vi "Dialog for DAQmx Configuration.vi"(6 "Variant":variant, 8 "error in":errorcluster, 11 "DAQmx config in":T4={"Run Mode"=0, "Sample Rate (Hz)"=51200.0, "Block Size"=5120, "Channel Table"=[], "Trigger Type"=0, "Trigger Channel"="", "Level"=0.0, "Pretrigger"=20, "Hysteresis"=0.0, "Slope"=enum."Rising"} {"Run Mode" items=["Run Once", "Continuously"]; "Block Size" min=0; "Sample Rate (Hz)" min=0.0; "Trigger Type" items=["None", "Analog Reference"]; "Channel Table"."input terminal configuration" items=["default"=-1, "RSE"=10083, "NRSE"=10078, "Differential"=10106, "Pseudodifferential"=12529]; "Channel Table"."Channel Type" items=["Voltage (V)"=0, "Charge (C)"=9, "-"=99, "SPL (Pa)"=3, "Force (lbf)"=6, "Force (N)"=1, "Acceleration (g) - IEPE"=2, "Acceleration (g) - Charge"=12, "Acceleration (g) - 4 wire DC Voltage"=22, "Velocity (in/s)"=7, "Velocity (mm/s)"=8, "Prox Probe (mil)"=4, "Prox Probe (mm)"=5]}) -> (0 "error out":errorcluster, 1 "Task Verified":T5, 3 "DAQmx config out":T4={"Run Mode"=0, "Sample Rate (Hz)"=51200.0, "Block Size"=5120, "Channel Table"=[], "Trigger Type"=0, "Trigger Channel"="", "Level"=0.0, "Pretrigger"=20, "Hysteresis"=0.0, "Slope"=enum."Rising"} {"Run Mode" items=["Run Once", "Continuously"]; "Block Size" min=0; "Sample Rate (Hz)" min=0.0; "Trigger Type" items=["None", "Analog Reference"]; "Channel Table"."input terminal configuration" items=["default"=-1, "RSE"=10083, "NRSE"=10078, "Differential"=10106, "Pseudodifferential"=12529]; "Channel Table"."Channel Type" items=["Voltage (V)"=0, "Charge (C)"=9, "-"=99, "SPL (Pa)"=3, "Force (lbf)"=6, "Force (N)"=1, "Acceleration (g) - IEPE"=2, "Acceleration (g) - Charge"=12, "Acceleration (g) - 4 wire DC Voltage"=22, "Velocity (in/s)"=7, "Velocity (mm/s)"=8, "Prox Probe (mil)"=4, "Prox Probe (mm)"=5]}, 4 "commit changes":bool)   [LabVIEW 2024, in "Dynamic Signal Acquisition (Interactive) UI.lvlib"]
doc: "Window Appearance = Dialog\n\nThis dialog configuration window reconfigures the DAQmx analog input task."
uses:
  Dynamic Signal Acquisition (Interactive) UI.lvlib
  SFPDAQmx Channel Info.ctl
  SFPDAQ Configuration.ctl
  <vilib>/addons/Sound and Vibration/svt_DAQmx/subVIs/Run Mode.ctl
  <vilib>/addons/Sound and Vibration/svt_DAQmx/subVIs/Verification Status.ctl
  <vilib>/addons/Sound and Vibration/svt_DAQmx/subVIs/Calibration and Reset Status.ctl
  <vilib>/Utility/miscctls.llb/LVPositionTypeDef.ctl
  <vilib>/addons/_NISVFA/_Shared subVIs/Controls/svc_Analog Level Trigger Configuration.ctl
  <vilib>/DAQmx/configure/task.llb/DAQmx Stop Task.vi
  <vilib>/addons/Sound and Vibration/svt_DAQmx/subVIs/Self Calibrate Devices (Dialog).vi
  <vilib>/Utility/cursorutil.llb/Set Busy.vi
  <vilib>/addons/Sound and Vibration/svt_DAQmx/subVIs/Reset Devices.vi
  <vilib>/Utility/cursorutil.llb/Unset Busy.vi
  <vilib>/DAQmx/configure/task.llb/DAQmx Control Task.vi
  <vilib>/addons/_NISVFA/_Shared subVIs/Common/svc_Clear Error Cluster for Specific Code.vi
  <vilib>/addons/Sound and Vibration/svt_DAQmx/subVIs/SV_DAQmx.lvlib
panel:
  in  "Run Mode":T1 items=["Once", "Continuously"]
  in  "Resolution":dbl=10.0 min=0.01 format="%_4g Hz"
  in  "Alias-Free Lines":i32=2000 min=2 max=4000000 step=1 format="%.0f lines"
  in  "Max Frequency":dbl=20000.0 min=0.0 format="%#_g Hz"
  in  "Block Duration":dbl=0.1 min=1e-06 max=100.0 format="%_4g s"
  in  "Block Size":i32=5120 min=2 max=10000000 step=1 format="%.0f samples"
  in  "Sample Rate":dbl=51200.0 min=0.0 format="%#_g Hz"
  in  "Channel Table":T2[](array[typedef]) {"input terminal configuration" items=["default"=-1, "RSE"=10083, "NRSE"=10078, "Differential"=10106, "Pseudodifferential"=12529]; "Channel Type" items=["Voltage (V)"=0, "Charge (C)"=9, "-"=99, "SPL (Pa)"=3, "Force (lbf)"=6, "Force (N)"=1, "Acceleration (g) - IEPE"=2, "Acceleration (g) - Charge"=12, "Acceleration (g) - 4 wire DC Voltage"=22, "Velocity (in/s)"=7, "Velocity (mm/s)"=8, "Prox Probe (mil)"=4, "Prox Probe (mm)"=5]}
  out "status string":string
  out "status":T3
  in  "Reset Devices":bool
  in  "Self Calibrate":bool
  in  "OK":bool
  in  "Error Details":bool
  in  "Cancel":bool
  in  "Slope":enum16{"Falling", "Rising"}(ring)=enum."Rising"
  in  "Hysteresis":dbl format="%#_g EU"
  in  "Pretrigger":i32=20 min=0 step=1 format="%.0f samples"
  in  "Level":dbl format="%#_g EU"
  in  "Channel":string(combo)
  in  "Enable SW Analog Ref Trig":bool
  # "Sampling Info"
  # "Channel Table"
  # "Physical Channel"
  # "Measurement Type"
  # "Range"
  # "mV/EU"
  # "Excitation"
  # "Coupling"
  # "Terminal Configuration"
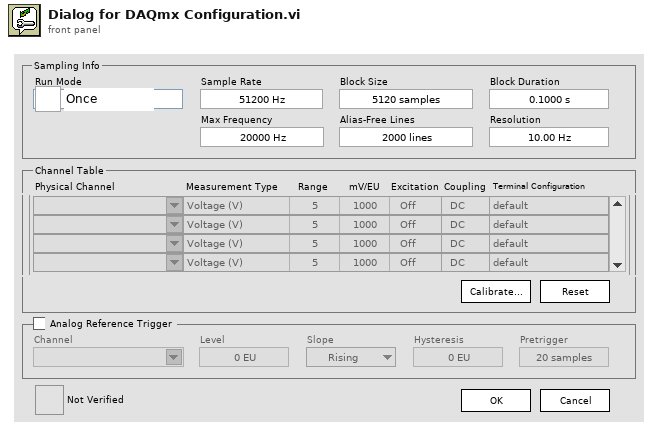
[diagram p1: front panel]
types:
  T1 = typedef "SV_DAQmx.lvlib/Run Mode.ctl" = u16
  T2 = typedef "Dynamic Signal Acquisition (Interactive) UI.lvlib/SFPDAQmx Channel Info.ctl" = cluster{"DAQmx Channel":tag, "Channel Type":u16, "Max":dbl, "Sensitivity":dbl, "Coupling":enum16{"AC", "DC"}, "input terminal configuration":i32, "excitation":enum16{"Off", "Min", "Max"}}
  T3 = typedef "SV_DAQmx.lvlib/Calibration and Reset Status.ctl" = u16
  T4 = typedef "Dynamic Signal Acquisition (Interactive) UI.lvlib/SFPDAQ Configuration.ctl" = cluster{"Run Mode":u16, "Sample Rate (Hz)":dbl, "Block Size":i32, "Channel Table":T2[], "Trigger Type":u16, "Trigger Channel":string, "Level":dbl, "Pretrigger":i32, "Hysteresis":dbl, "Slope":enum16{"Falling", "Rising"}}
  T5 = typedef "SV_DAQmx.lvlib/Verification Status.ctl" = bool
  T6 = enum32{"Invalid", "Standard", "Closed", "Hidden", "Minimized", "Maximized"}
  T7 = typedef "LVPositionTypeDef.ctl" = cluster{"Left":i32, "Top":i32}
  T8 = typedef "LVRectTypeDef.ctl" = cluster{"Left":i16, "Top":i16, "Right":i16, "Bottom":i16}
  T9 = enum8{"Enabled", "Disabled", "Disabled and Grayed Out"}
  T10 = typedef "svc_Analog Level Trigger Configuration.ctl" = cluster{"level":dbl, "slope":u16, "hysteresis":dbl}
  T11 = cluster{"enable":bool, "channel":string, "level trigger configuration":T10, "pretrigger":i32}
  T12 = cluster{"Shift":bool, "Ctrl":bool, "Alt":bool, "Cmd":bool, "Opt":bool}
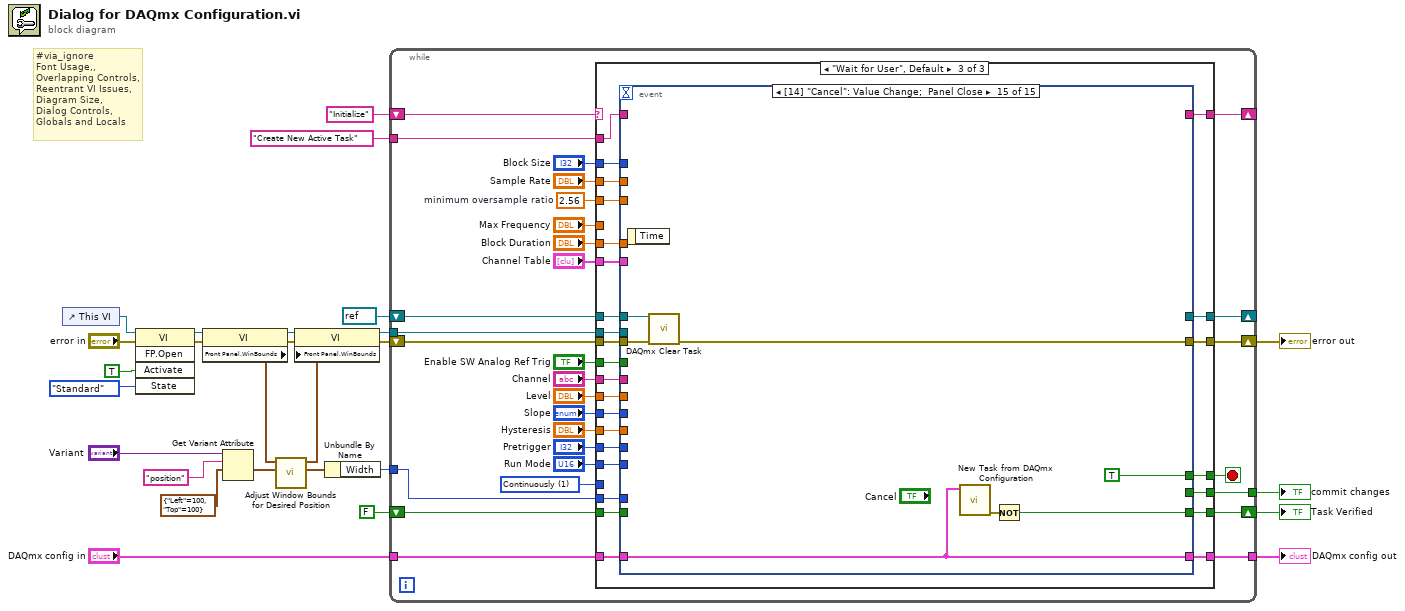
[diagram p0: block diagram]
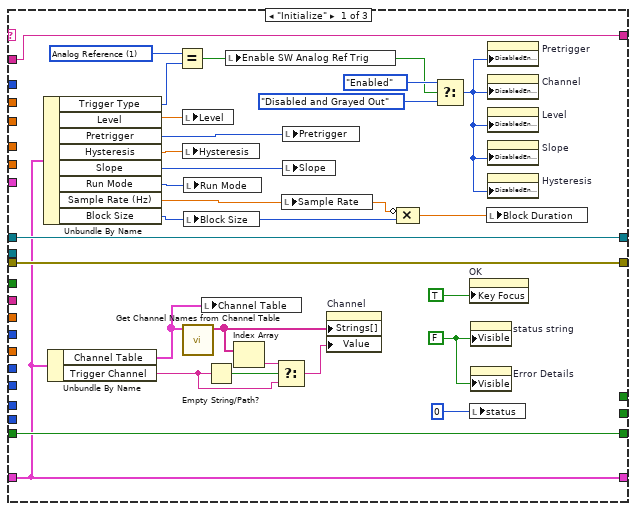
[diagram p2: hidden frame]
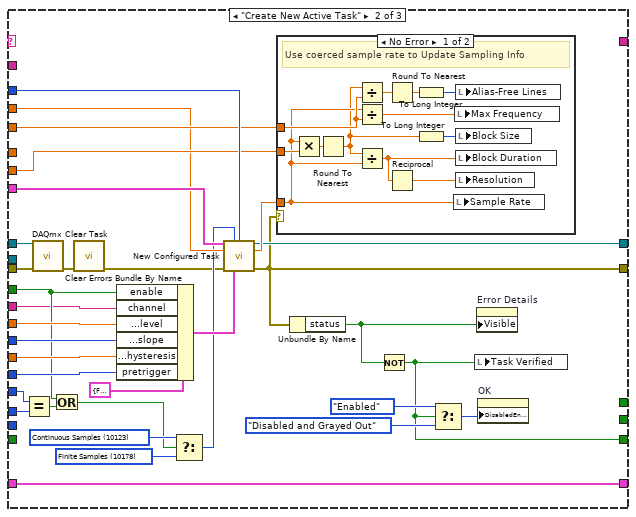
[diagram p3: hidden frame]
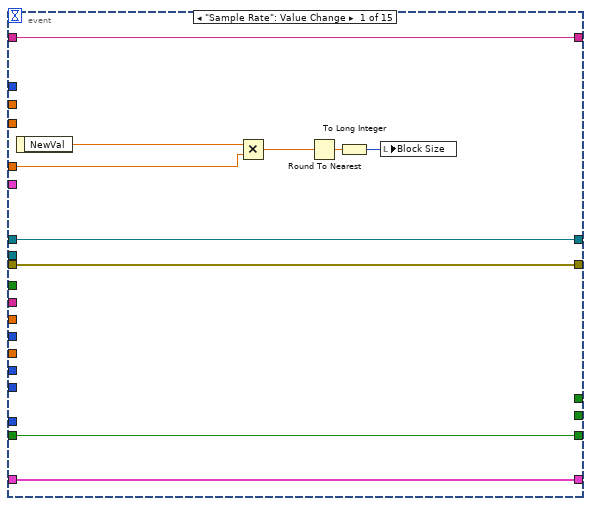
[diagram p5: hidden frame]
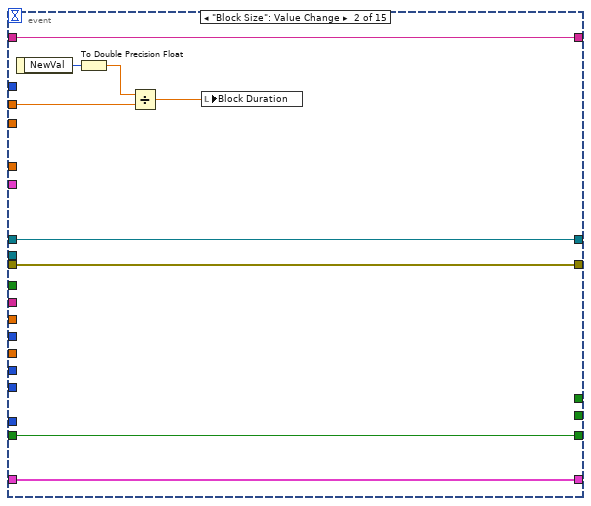
[diagram p6: hidden frame]
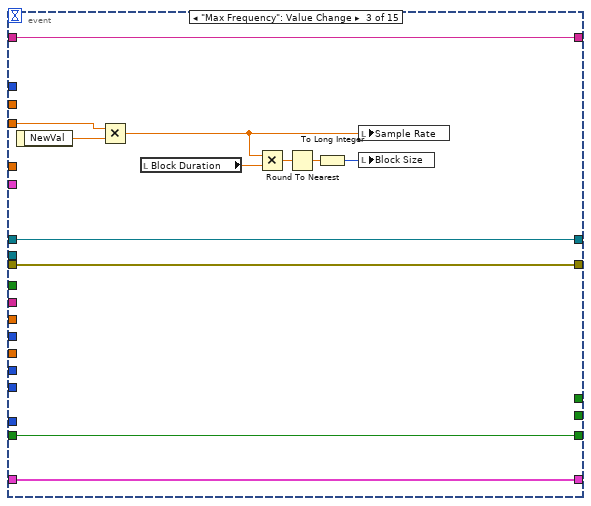
[diagram p7: hidden frame]
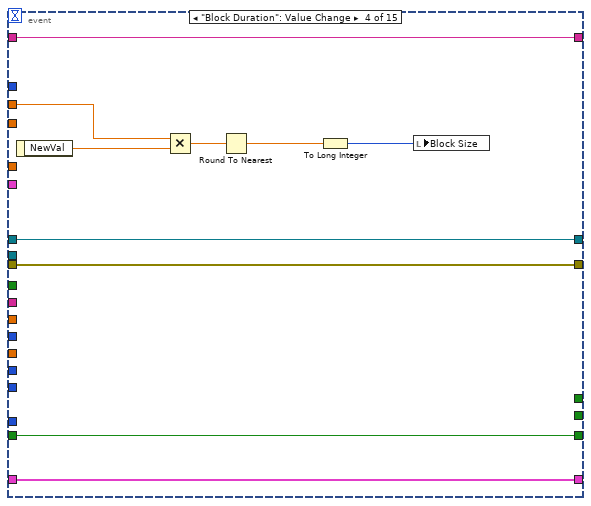
[diagram p8: hidden frame]
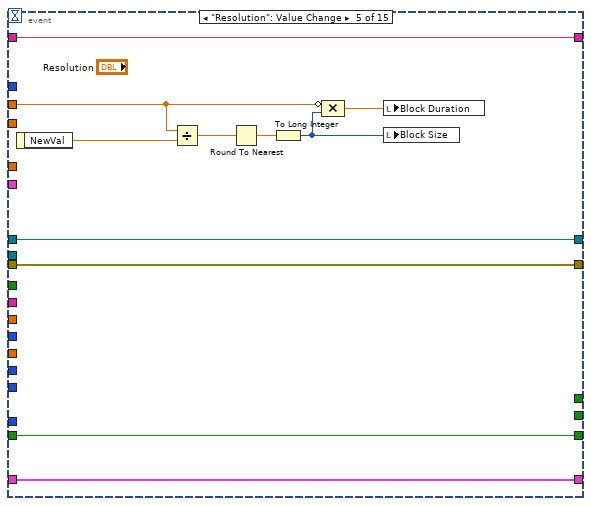
[diagram p9: hidden frame]
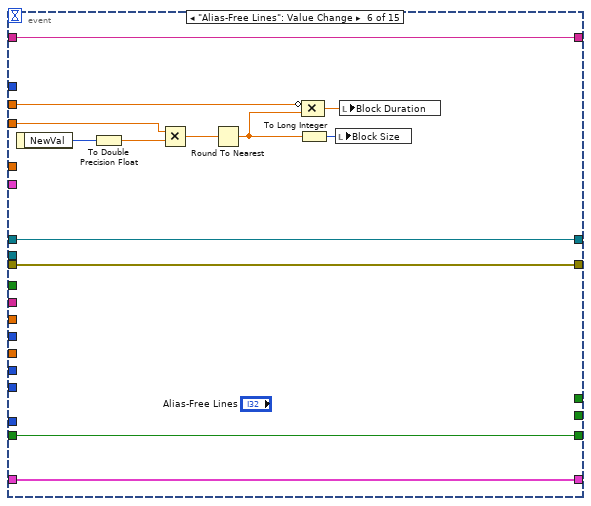
[diagram p10: hidden frame]
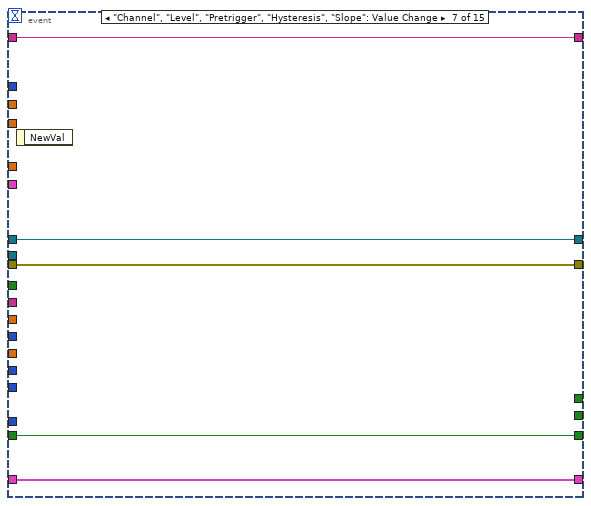
[diagram p11: hidden frame]
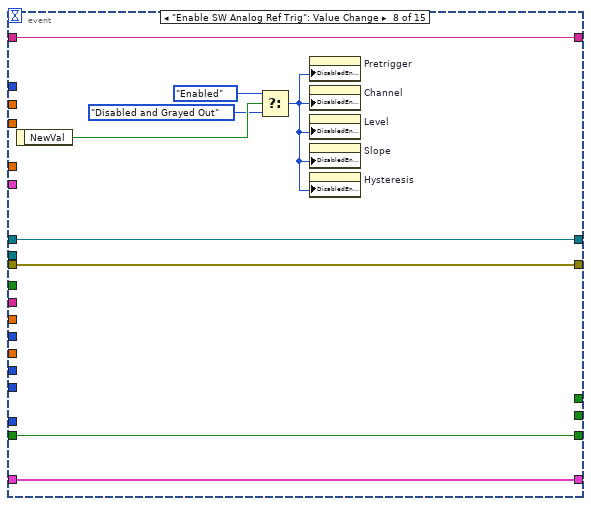
[diagram p12: hidden frame]
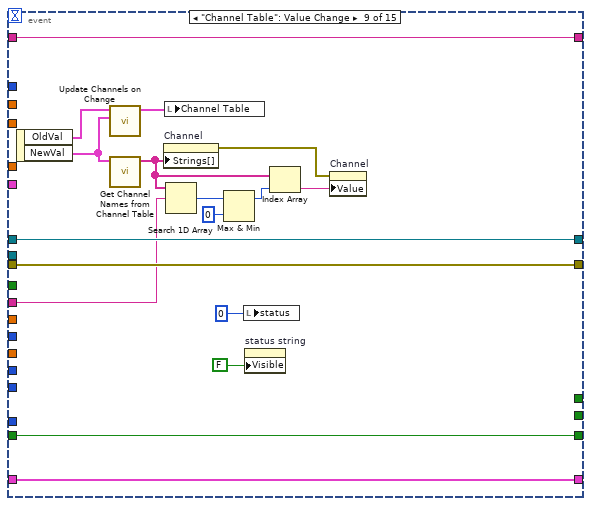
[diagram p13: hidden frame]
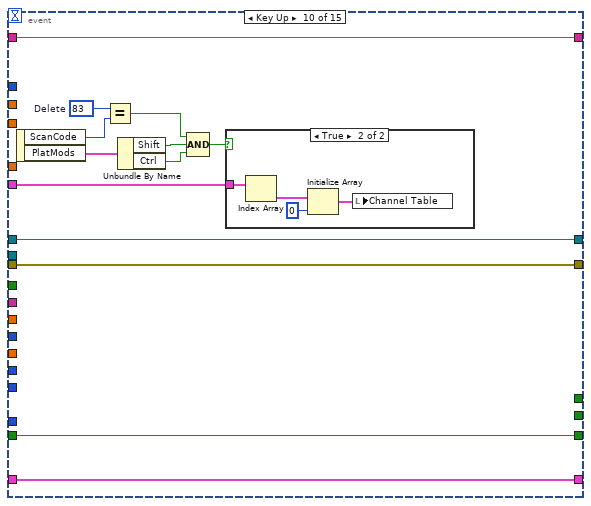
[diagram p14: hidden frame]
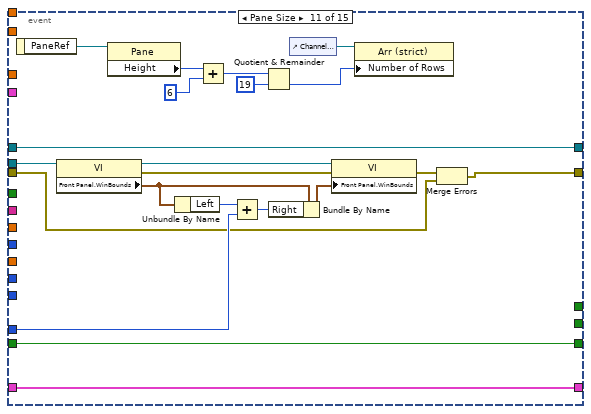
[diagram p16: hidden frame]
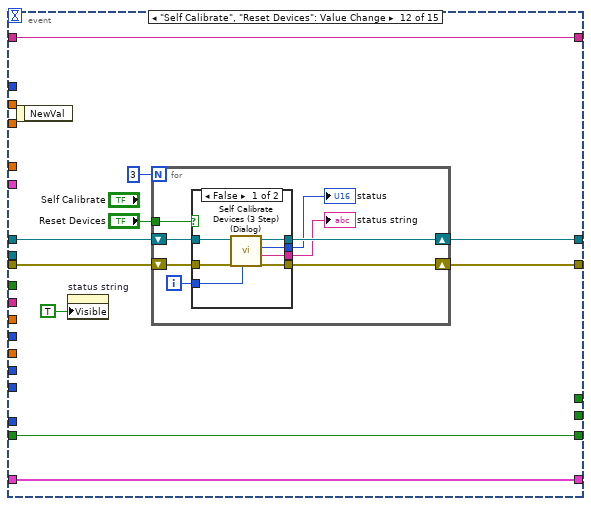
[diagram p17: hidden frame]
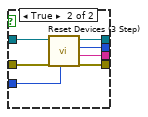
[diagram p18: hidden frame]
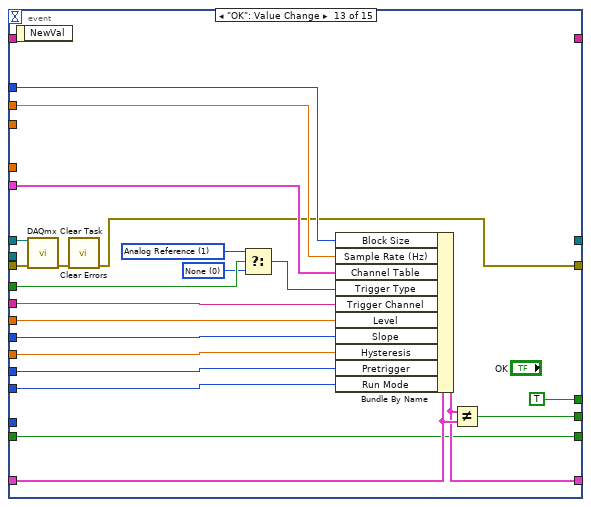
[diagram p19: hidden frame]
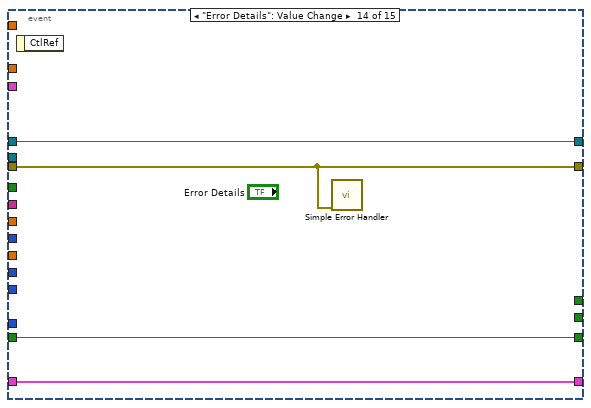
[diagram p20: hidden frame]
diagram:
  # "#via_ignore  \nFont Usage,,\nOverlapping Controls,\nReentrant VI Issues,\nDiagram Size,\nDialog Controls,\nGlobals and Locals"
  n1 = control-ref of="This VI"() -> (w2:refnum<vi>)
  n2 = invoke on="Invoke Node" class="VI" method="FP.Open"(reference=w2, error in="error in", "Activate"=TRUE ("Activate?"), "State"=T6."Standard") -> (reference out=w14:refnum<vi>, error out=w13:errorcluster)  [unwired: 1 in, 3 out]
  n3 = property on="Property Node" class="VI"(reference=w14, error in=w13) -> (reference out=w24:refnum<vi>, error out=w23:errorcluster, "Front Panel.WinBounds"=w22:T8)
  n4 = Get Variant Attribute(Variant="Variant", name="position" ("f"), default value (empty Variant)=T7 {"Left"=100, "Top"=100} ("Position")) -> (value=w17:T7)  [unwired: 1 in, 3 out]
  n5 = call "Adjust Window Bounds for Desired Position.vi"("Position"=w17, "Front Panel.WinBounds in"=w22) -> ("Dimensions"=w8:cluster{"Width":i16, "Height":i16}, "Front Panel.WinBounds out"=w20:T8)  [unwired: 8 in]
  n6 = property on="Property Node" class="VI"(reference=w24, error in=w23, "Front Panel.WinBounds"=w20) -> (reference out=w10:refnum<vi>, error out=w21:errorcluster)
  n7 = Unbundle By Name(w8) -> ("Width"=w7:i16)
  n8 = while {
    shift-right: [w56] -> _
    shift-left: refnum<k21> refnum ("task in") -> [w55]
    shift-right: [w37] -> _
    shift-left: "Initialize" ("Sampling Info") -> [w29]
    shift-right: [w53] -> w3
    shift-left: w21 -> [w54]
    tunnel: "DAQmx config in" -> [w52]
    tunnel: [w51] -> w1
    shift-right: [w38] -> w12
    shift-left: FALSE -> [w39]
    tunnel: [w36] -> w25
    tunnel: w10 -> [w32]
    tunnel: w7 -> [w31]
    tunnel: "Create New Active Task" ("Sampling Info") -> [w30]
    stop <- w28 stop-if-true
    w35 = T1 1 items=["Once", "Continuously"] ("Run Mode")
    w40 = 2.56  # minimum oversample ratio
    n9 = case shown="\"Wait for User\", Default" w29 {
      tunnel: [w67 w107 w141] -> w56
      tunnel: w55 -> [w67 w87 w142]
      tunnel: w54 -> [w84 w86 w140]
      tunnel: [w84 w91 w139] -> w53
      tunnel: w52 -> [w66 w117 w155]
      tunnel: [w66 w117 w154] -> w51
      tunnel: "Channel Table" -> [_ w103 w150]
      tunnel: "Enable SW Analog Ref Trig" -> [_ w98 w148]
      tunnel: "Channel" -> [_ w96 w149]
      tunnel: "Level" -> [_ w106 w147]
      tunnel: "Slope" -> [_ w105 w145]
      tunnel: "Pretrigger" -> [_ w101 w146]
      tunnel: "Hysteresis" -> [_ w104 w144]
      tunnel: "Sample Rate" -> [_ w99 w151]
      tunnel: "Block Size" -> [_ w116 w152]
      tunnel: "Run Mode" -> [_ w112 w143]
      tunnel: w35 -> [_ w111 _]
      tunnel: [_ _ w153] -> w28
      tunnel: w40 -> [_ w109 w138]
      tunnel: [w83 w92 w136] -> w38
      tunnel: w39 -> [w83 _ w137]
      tunnel: [w59 _ w131] -> w37
      tunnel: [_ _ w135] -> w36
      tunnel: "Max Frequency" -> [_ _ _]
      tunnel: "Block Duration" -> [_ w108 w134]
      tunnel: w32 -> [_ _ w133]
      tunnel: w31 -> [_ _ w132]
      tunnel: w30 -> [w59 _ w130]
      frame "Initialize" {
        w62 = FALSE ("Visible")
        w75 = u16 1 items=["None", "Analog Reference"] ("Trigger Type")
        n10 = Unbundle By Name(w66) -> ("Trigger Type"=w74:u16, "Level"=w76:dbl, "Pretrigger"=w77:i32, "Hysteresis"=w78:dbl, "Slope"=w79:enum16{"Falling", "Rising"}, "Run Mode"=w80:u16, "Sample Rate (Hz)"=w58:dbl, "Block Size"=w57:i32)
        n11 = Unbundle By Name(w66) -> ("Channel Table"=w65:T2[], "Trigger Channel"=w64:string)
        n12 = Equal?(x=w75, y=w74) -> (x = y?=w70:bool)
        n13 = local write "Level"(w76) -> ()
        n14 = local write "Hysteresis"(w78) -> ()
        n15 = call "Get Channel Names from Channel Table.vi"("Channel Table"=w65) -> ("All Channels"=w69:string[])  [unwired: 10 in]
        n16 = local write "Run Mode"(w80) -> ()
        n17 = local write "Block Size"(w57) -> ()
        n18 = local write "Channel Table"(w65) -> ()
        n19 = Empty String/Path?(string/path=w64) -> (empty?=w82:bool)
        n20 = local write "Enable SW Analog Ref Trig"(w70) -> ()
        n21 = Index Array(array=w69) -> (element=w68:string)  [unwired: 1 in]
        n22 = Select(t=w68, s=w82, f=w64) -> (s? t:f=w81:string)
        n23 = local write "Sample Rate"(w58) -> ()
        n24 = local write "Pretrigger"(w77) -> ()
        n25 = local write "Slope"(w79) -> ()
        n26 = property on="Channel" class="CmbBox"("Strings[]"=w69, "Value"=w81) -> ()  [unwired: 2 in, 2 out]
        n27 = Compound Arithmetic op=MULTIPLY(invert w58, w57) -> (w63:dbl)
        n28 = Select(t=T9."Enabled" ("Disabled"), s=w70, f=T9."Disabled and Grayed Out") -> (s? t:f=w71:T9)
        n29 = property on="OK" class="Bool"("Key Focus"=TRUE) -> ()  [unwired: 2 in, 2 out]
        n30 = local write "status"(u16 0 ("status")) -> ()
        n31 = property on="status string" class="Str"("Visible"=w62) -> ()  [unwired: 2 in, 2 out]
        n32 = property on="Error Details" class="Bool"("Visible"=w62) -> ()  [unwired: 2 in, 2 out]
        n33 = local write "Block Duration"(w63) -> ()
        n34 = property on="Pretrigger" class="DigNum (strict)"("DisabledEnum"=w71) -> ()  [unwired: 2 in, 2 out]
        n35 = property on="Channel" class="CmbBox"("DisabledEnum"=w71) -> ()  [unwired: 2 in, 2 out]
        n36 = property on="Level" class="DigNum (strict)"("DisabledEnum"=w71) -> ()  [unwired: 2 in, 2 out]
        n37 = property on="Slope" class="Enum (strict)"("DisabledEnum"=w71) -> ()  [unwired: 2 in, 2 out]
        n38 = property on="Hysteresis" class="DigNum (strict)"("DisabledEnum"=w71) -> ()  [unwired: 2 in, 2 out]
      }
      frame "Create New Active Task" {
        w114 = 10178 items=["Finite Samples"=10178, "Continuous Samples"=10123, "Hardware Timed Single Point"=12522] ("sample mode")
        w113 = 10123 items=["Finite Samples"=10178, "Continuous Samples"=10123, "Hardware Timed Single Point"=12522] ("sample mode")
        n39 = Equal?(x=w112, y=w111) -> (x = y?=w115:bool)
        n40 = call <vilib>:"DAQmx Clear Task.vi"("task in"=w87, "error in"=w86) -> ("error out"=w88:errorcluster)  [unwired: 13 in]
        n41 = Or(x=w98, y=w115) -> (x .or. y?=w89:bool)
        n42 = call <vilib>:"Clear Errors.vi"("error in (no error)"=w88) -> ("error out"=w85:errorcluster)  [unwired: 5 in, 1 out]
        n43 = Bundle By Name(cluster=T11 {"enable"=FALSE, "channel"="", "level trigger configuration"={"level"=0.0, "slope"=0, "hysteresis"=0.0}, "pretrigger"=0} ("analog reference trigger configuration"), "enable"=w98, "channel"=w96, "level trigger configuration.level"=w106, "level trigger configuration.slope"=w105, "level trigger configuration.hysteresis"=w104, "pretrigger"=w101) -> (w100:T11)
        n44 = Select(t=w113, s=w89, f=w114) -> (s? t:f=w97:i32)
        n45 = call "New Configured Task.vi"("channel table"=w103, "sample mode"=w97, "block size"=w116, "sample rate"=w99, "error in"=w85, "analog reference trigger configuration"=w100) -> ("DAQmx analog input task"=w107:refnum<k21>, "actual sample rate"=w110:dbl, "error out"=w91:errorcluster)  [unwired: 7 in]
        n46 = case shown="No Error" w91 {
          tunnel: w110 -> [w120 _]
          tunnel: w109 -> [w122 _]
          tunnel: w108 -> [w121 _]
          frame No Error {
            # "Use coerced sample rate to Update Sampling Info"
            n47 = Multiply(x=w120, y=w121) -> (x*y=w123:dbl)
            n48 = Round To Nearest(number=w123) -> (nearest integer value=w119:dbl)
            n49 = Divide(x=w119, y=w122) -> (x/y=w127:dbl)
            n50 = Divide(x=w120, y=w122) -> (x/y=w124:dbl)
            n51 = Divide(x=w119, y=w120) -> (x/y=w128:dbl)
            n52 = Round To Nearest(number=w127) -> (nearest integer value=w126:dbl)
            n53 = Reciprocal(x=w128) -> (1/x=w129:dbl)
            n54 = To Long Integer(number=w126) -> (32bit integer=w125:i32)
            n55 = To Long Integer(number=w119) -> (32bit integer=w118:i32)
            n56 = local write "Sample Rate"(w120) -> ()
            n57 = local write "Max Frequency"(w124) -> ()
            n58 = local write "Alias-Free Lines"(w125) -> ()
            n59 = local write "Block Size"(w118) -> ()
            n60 = local write "Block Duration"(w128) -> ()
            n61 = local write "Resolution"(w129) -> ()
          }
          frame Error {
          }
        }
        n62 = Unbundle By Name(w91) -> ("status"=w90:bool)
        n63 = Not(x=w90) -> (.not. x?=w92:bool)
        n64 = Select(t=T9."Enabled" ("Disabled"), s=w92, f=T9."Disabled and Grayed Out" ("Disabled")) -> (s? t:f=w95:T9)
        n65 = local write "Task Verified"(w92) -> ()
        n66 = property on="Error Details" class="Bool"("Visible"=w90) -> ()  [unwired: 2 in, 2 out]
        n67 = property on="OK" class="Bool"("DisabledEnum"=w95) -> ()  [unwired: 2 in, 2 out]
      }
      frame "Wait for User", Default {
        n68 = event shown="[14] \"Cancel\": Value Change;  Panel Close" {
          selector: _ -> [_ _ _ _ _ _ _ _ _ _ _ _ _ _ _]
          dyn-events: _ -> [_ _ _ _ _ _ _ _ _ _ _ _ _ _ _]
          timeout: _ -> [_ _ _ _ _ _ _ _ _ _ _ _ _ _ _]
          tunnel: w155 -> [w165 w174 w186 w196 w207 w220 w225 w234 w251 w264 w289 w299 w332 w347 w352]
          tunnel: [w165 w174 w186 w196 w207 w220 w225 w234 w251 w264 w289 w299 w327 w347 w352] -> w154
          tunnel: [_ _ _ _ _ _ _ _ _ _ _ _ TRUE _ TRUE] -> w153
          tunnel: w152 -> [_ _ _ _ _ _ _ _ _ _ _ _ w343 _ _]
          tunnel: w151 -> [_ w170 _ w188 w197 w213 _ _ _ _ _ _ w342 _ _]
          tunnel: w150 -> [_ _ _ _ _ _ _ _ _ w253 _ _ w341 _ _]
          tunnel: w149 -> [_ _ _ _ _ _ _ _ w248 _ _ _ w328 _ _]
          tunnel: w148 -> [_ _ _ _ _ _ _ _ _ _ _ _ w340 _ _]
          tunnel: w147 -> [_ _ _ _ _ _ _ _ _ _ _ _ w336 _ _]
          tunnel: w146 -> [_ _ _ _ _ _ _ _ _ _ _ _ w329 _ _]
          tunnel: w145 -> [_ _ _ _ _ _ _ _ _ _ _ _ w335 _ _]
          tunnel: w144 -> [_ _ _ _ _ _ _ _ _ _ _ _ w334 _ _]
          tunnel: w143 -> [_ _ _ _ _ _ _ _ _ _ _ _ w333 _ _]
          tunnel: w142 -> [w164 w173 w185 w195 w205 w218 w223 w232 w249 w262 w288 w297 w325 w346 w350]
          tunnel: w140 -> [w163 w172 w184 w194 w206 w219 w224 w233 w250 w263 w271 w295 w324 w344 w351]
          tunnel: [w163 w172 w184 w194 w206 w219 w224 w233 w250 w263 w269 w291 w322 w344 w353] -> w139
          tunnel: [w164 w173 w185 w195 w205 w218 w223 w232 w249 w262 w288 w296 _ w346 _] -> w141
          tunnel: w138 -> [_ _ w182 _ _ w217 _ _ _ _ _ _ _ _ _]
          tunnel: w137 -> [w162 w171 w181 w189 w202 w214 w222 w231 w247 w261 w287 w298 w326 w345 _]
          tunnel: [w162 w171 w181 w189 w202 w214 w222 w231 w247 w261 w287 w298 w326 w345 w348] -> w136
          tunnel: [_ _ _ _ _ _ _ _ _ _ _ _ w331 _ _] -> w135
          tunnel: w134 -> [w157 _ _ _ _ _ _ _ _ _ _ _ _ _ _]
          tunnel: w133 -> [_ _ _ _ _ _ _ _ _ _ w274 _ _ _ _]
          tunnel: w132 -> [_ _ _ _ _ _ _ _ _ _ w273 _ _ _ _]
          tunnel: [w156 w167 w175 w187 w198 w209 w221 w226 w239 w252 _ w293 _ _ _] -> w131
          tunnel: w130 -> [w156 w167 w175 w187 w198 w209 w221 w226 w239 w252 _ w293 _ _ _]
          event "Sample Rate": Value Change {
            n69 = event-data() -> ("NewVal"=w161:dbl)  [unwired: 1 in]
            n70 = Multiply(x=w161, y=w157) -> (x*y=w160:dbl)
            n71 = Round To Nearest(number=w160) -> (nearest integer value=w159:dbl)
            n72 = To Long Integer(number=w159) -> (32bit integer=w158:i32)
            n73 = local write "Block Size"(w158) -> ()
          }
          event "Block Size": Value Change {
            n74 = event-data() -> ("NewVal"=w168:i32)  [unwired: 1 in]
            n75 = To Double Precision Float(number=w168) -> (double precision float=w166:dbl)
            n76 = Divide(x=w166, y=w170) -> (x/y=w169:dbl)
            n77 = local write "Block Duration"(w169) -> ()
          }
          event "Max Frequency": Value Change {
            n78 = event-data() -> ("NewVal"=w183:dbl)  [unwired: 1 in]
            n79 = Multiply(x=w182, y=w183) -> (x*y=w176:dbl)
            n80 = local read "Block Duration"() -> (w180:dbl)
            n81 = Multiply(x=w176, y=w180) -> (x*y=w179:dbl)
            n82 = Round To Nearest(number=w179) -> (nearest integer value=w178:dbl)
            n83 = To Long Integer(number=w178) -> (32bit integer=w177:i32)
            n84 = local write "Sample Rate"(w176) -> ()
            n85 = local write "Block Size"(w177) -> ()
          }
          event "Block Duration": Value Change {
            n86 = event-data() -> ("NewVal"=w193:dbl)  [unwired: 1 in]
            n87 = Multiply(x=w188, y=w193) -> (x*y=w192:dbl)
            n88 = Round To Nearest(number=w192) -> (nearest integer value=w190:dbl)
            n89 = To Long Integer(number=w190) -> (32bit integer=w191:i32)
            n90 = local write "Block Size"(w191) -> ()
          }
          event "Resolution": Value Change {
            n91 = event-data() -> ("NewVal"=w201:dbl)  [unwired: 1 in]
            n92 = Divide(x=w197, y=w201) -> (x/y=w204:dbl)
            n93 = Round To Nearest(number=w204) -> (nearest integer value=w203:dbl)
            n94 = To Long Integer(number=w203) -> (32bit integer=w200:i32)
            n95 = Compound Arithmetic op=MULTIPLY(invert w197, w200) -> (w199:dbl)
            n96 = local write "Block Duration"(w199) -> ()
            n97 = local write "Block Size"(w200) -> ()
          }
          event "Alias-Free Lines": Value Change {
            n98 = event-data() -> ("NewVal"=w216:i32)  [unwired: 1 in]
            n99 = To Double Precision Float(number=w216) -> (double precision float=w208:dbl)
            n100 = Multiply(x=w217, y=w208) -> (x*y=w215:dbl)
            n101 = Round To Nearest(number=w215) -> (nearest integer value=w211:dbl)
            n102 = To Long Integer(number=w211) -> (32bit integer=w212:i32)
            n103 = Compound Arithmetic op=MULTIPLY(invert w213, w211) -> (w210:dbl)
            n104 = local write "Block Size"(w212) -> ()
            n105 = local write "Block Duration"(w210) -> ()
          }
          event "Channel", "Level", "Pretrigger", "Hysteresis", "Slope": Value Change {
            n106 = event-data() -> ()  [unwired: 1 in, 1 out]
          }
          event "Enable SW Analog Ref Trig": Value Change {
            n107 = event-data() -> ("NewVal"=w230:bool)  [unwired: 1 in]
            n108 = Select(t=T9."Enabled" ("Disabled"), s=w230, f=T9."Disabled and Grayed Out") -> (s? t:f=w228:T9)
            n109 = property on="Pretrigger" class="DigNum (strict)"("DisabledEnum"=w228) -> ()  [unwired: 2 in, 2 out]
            n110 = property on="Channel" class="CmbBox"("DisabledEnum"=w228) -> ()  [unwired: 2 in, 2 out]
            n111 = property on="Level" class="DigNum (strict)"("DisabledEnum"=w228) -> ()  [unwired: 2 in, 2 out]
            n112 = property on="Slope" class="Enum (strict)"("DisabledEnum"=w228) -> ()  [unwired: 2 in, 2 out]
            n113 = property on="Hysteresis" class="DigNum (strict)"("DisabledEnum"=w228) -> ()  [unwired: 2 in, 2 out]
          }
          event "Channel Table": Value Change {
            n114 = event-data() -> ("OldVal"=w244:T2[], "NewVal"=w243:T2[])  [unwired: 1 in]
            n115 = call "Update Channels on Change.vi"("new channel table"=w243, "old channel table"=w244) -> ("updated channel table"=w245:T2[])  [unwired: 9 in]
            n116 = call "Get Channel Names from Channel Table.vi"("Channel Table"=w243) -> ("All Channels"=w246:string[])  [unwired: 10 in]
            n117 = property on="Channel" class="CmbBox"("Strings[]"=w246) -> (error out=w242:errorcluster)  [unwired: 2 in, 1 out]
            n118 = local write "Channel Table"(w245) -> ()
            n119 = Search 1D Array(1D array=w246, element=w248) -> (index of element=w236:i32)  [unwired: 1 in]
            n120 = Max & Min(x=w236, y=0) -> (max(x,y)=w237:i32)  [unwired: 1 out]
            n121 = local write "status"(u16 0 ("status")) -> ()
            n122 = property on="status string" class="Str"("Visible"=FALSE) -> ()  [unwired: 2 in, 2 out]
            n123 = Index Array(array=w246, index=w237) -> (element=w238:string)
            n124 = property on="Channel" class="CmbBox"(error in=w242, "Value"=w238) -> ()  [unwired: 1 in, 2 out]
          }
          event Key Up {
            w256 = i16 83  # Delete
            n125 = event-data() -> ("ScanCode"=w257:i16, "PlatMods"=w260:T12)  [unwired: 1 in]
            n126 = Equal?(x=w256, y=w257) -> (x = y?=w255:bool)
            n127 = Unbundle By Name(w260) -> ("Shift"=w259:bool, "Ctrl"=w258:bool)
            n128 = Compound Arithmetic op=AND(w255, w259, w258) -> (w254:bool)
            n129 = case shown="True" w254 {
              tunnel: w253 -> [_ w267]
              frame False {
              }
              frame True {
                n130 = Index Array(array=w267) -> (element=w266:T2)  [unwired: 1 in]
                n131 = Initialize Array(w266, 0 ("dimension size")) -> (w265:T2[])
                n132 = local write "Channel Table"(w265) -> ()
              }
            }
          }
          event Pane Size {
            n133 = event-data() -> ("PaneRef"=w286:refnum<vi>)  [unwired: 1 in]
            n134 = property on="Property Node" class="VI"(reference=w274) -> (reference out=w275:refnum<vi>, error out=w276:errorcluster, "Front Panel.WinBounds"=w277:T8)  [unwired: 1 in]
            n135 = property on="Property Node" class="Pane"(reference=w286) -> ("Height"=w284:u32)  [unwired: 1 in, 2 out]
            n136 = Unbundle By Name(w277) -> ("Left"=w272:i16)
            n137 = Add(x=w284, y=u32 6) -> (x+y=w281:u32)
            n138 = Add(x=w272, y=w273) -> (x+y=w278:i16)
            n139 = Quotient & Remainder(x=w281, y=u32 19) -> (floor(x/y)=w282:u32)  [unwired: 1 out]
            n140 = Bundle By Name(cluster=w277, "Right"=w278) -> (w279:T8)
            n141 = control-ref of="Channel Table"() -> (w285:refnum<vi>)
            n142 = property on="Property Node" class="VI"(reference=w275, error in=w276, "Front Panel.WinBounds"=w279) -> (error out=w270:errorcluster)  [unwired: 1 out]
            n143 = property on="Property Node" class="Arr (strict)"(reference=w285, "Number of Rows"=w282) -> ()  [unwired: 1 in, 2 out]
            n144 = Merge Errors(w270, w271) -> (w269:errorcluster)
          }
          event "Self Calibrate", "Reset Devices": Value Change {
            n145 = event-data() -> ()  [unwired: 1 in, 1 out]
            n146 = property on="status string" class="Str"("Visible"=TRUE) -> ()  [unwired: 2 in, 2 out]
            n147 = for {
              N: 3 -> [_]
              shift-right: [w306] -> w296
              shift-left: w297 -> [w307]
              shift-right: [w304] -> w291
              shift-left: w295 -> [w305]
              tunnel: "Reset Devices" -> [w300]
              i -> [w303]
              n148 = case shown="False" w300 {
                tunnel: w307 -> [w314 w321]
                tunnel: [w313 w315] -> w306
                tunnel: w305 -> [w312 w320]
                tunnel: [w311 w318] -> w304
                tunnel: [w310 w316] -> w301
                tunnel: [w309 w317] -> w302
                tunnel: w303 -> [w308 w319]
                frame False {
                  n149 = call <vilib>:"Self Calibrate Devices (3 Step) (Dialog).vi"("step"=w308, "error in"=w312, "task in"=w314) -> ("error out"=w311:errorcluster, "status string"=w309:string, "status"=w310:T3, "task out"=w313:refnum<k21>)  [unwired: 5 in]
                }
                frame True {
                  n150 = call <vilib>:"Reset Devices (3 Step).vi"("step"=w319, "error in"=w320, "task in"=w321) -> ("error out"=w318:errorcluster, "status string"=w317:string, "status"=w316:T3, "task out"=w315:refnum<k21>)  [unwired: 4 in, 1 out]
                }
              }
              "status string" <- w302
              "status" <- w301
            }
          }
          event "OK": Value Change {
            w339 = u16 0 items=["None", "Analog Reference"] ("Trigger Type")
            w338 = u16 1 items=["None", "Analog Reference"] ("Trigger Type")
            n151 = event-data() -> ()  [unwired: 1 in, 1 out]
            n152 = call <vilib>:"DAQmx Clear Task.vi"("task in"=w325, "error in"=w324) -> ("error out"=w323:errorcluster)  [unwired: 13 in]
            n153 = call <vilib>:"Clear Errors.vi"("error in (no error)"=w323) -> ("error out"=w322:errorcluster)  [unwired: 5 in, 1 out]
            n154 = Select(t=w338, s=w340, f=w339) -> (s? t:f=w337:u16)
            n155 = Bundle By Name(cluster=w332, "Block Size"=w343, "Sample Rate (Hz)"=w342, "Channel Table"=w341, "Trigger Type"=w337, "Trigger Channel"=w328, "Level"=w336, "Slope"=w335, "Hysteresis"=w334, "Pretrigger"=w329, "Run Mode"=w333) -> (w327:T4)
            n156 = Not Equal?(x=w327, y=w332) -> (x != y?=w331:bool)
          }
          event "Error Details": Value Change {
            n157 = event-data() -> ()  [unwired: 1 in, 1 out]
            n158 = call <vilib>:"Simple Error Handler.vi"("error in (no error)"=w344) -> ()  [unwired: 4 in, 5 out]
          }
          event "Cancel": Value Change; Panel Close {
            n159 = event-data() -> ()  [unwired: 1 in, 1 out]
            n160 = call <vilib>:"DAQmx Clear Task.vi"("task in"=w350, "error in"=w351) -> ("error out"=w353:errorcluster)  [unwired: 13 in]
            n161 = call "New Task from DAQmx Configuration.vi"("DAQmx Cfg"=w352) -> ("error out"=w349:errorcluster)  [unwired: 9 in, 1 out]
            n162 = Not(x=w349) -> (.not. x?=w348:bool)
          }
        }
      }
    }
  }
  "error out" <- w3
  "DAQmx config out" <- w1
  "Task Verified" <- w12
  "commit changes" <- w25
